vi "test Import Error when No Channels.vi"(8 "error in":errorcluster, 11 "TestCase in":refnum<class "1553 Parameters Import.lvclass">) -> (0 "error out":errorcluster, 3 "TestCase out":refnum<class "1553 Parameters Import.lvclass">)   [LabVIEW 2020, in "1553 Parameters Import.lvclass"]
uses:
  1553 Parameters Import.lvclass
  Shared/BIU Configuration.ctl
  Shared/Address.ctl
  Shared/Major Frame Definition.ctl
  Shared/Minor Frame Definition.ctl
  Shared/Acyclic Frame Definition.ctl
  Shared/Message Definition.ctl
  Shared/Message Type.ctl
  Shared/Terminal Endpoint.ctl
  Shared/Parameter Definition.ctl
  <vilib>/Utility/xml.llb/Write to XML File(string).vi
  <vilib>/addons/_JKI Toolkits/VI Tester/TestCase.llb/TestCase.lvclass
  Import/MIL-STD 1553 Import.lvlib
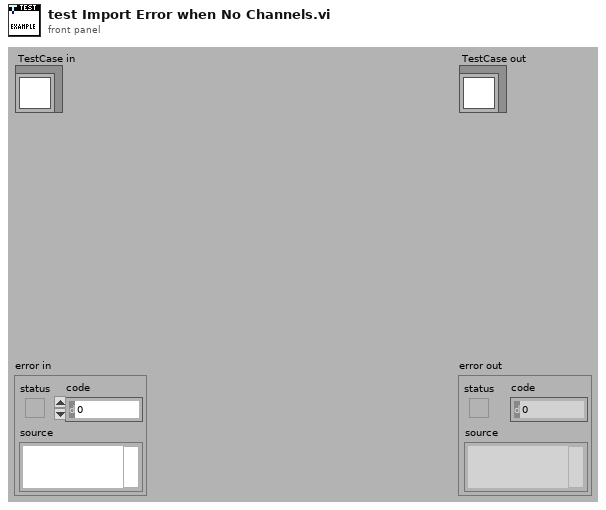
[diagram p1: front panel]
types:
  T1 = typedef "BIU Configuration.ctl" = cluster{"HW channel":u16, "terminal addresses":T2[], "terminal names":string[], "major frames":T3[], "minor frames":T4[], "acyclic frames":T5[], "messages":T6[], "minor frame period (us)":i32}
  T2 = typedef "Address.ctl" = u16
  T3 = typedef "Major Frame Definition.ctl" = cluster{"name":string, "minor frames":string[]}
  T4 = typedef "Minor Frame Definition.ctl" = cluster{"name":string, "messages":string[]}
  T5 = typedef "Acyclic Frame Definition.ctl" = cluster{"name":string, "messages":string[]}
  T6 = typedef "Message Definition.ctl" = cluster{"name":string, "message type":T7, "endpoint Tx":T8, "endpoint Rx":T8, "create timestamp channel":bool, "mode code":u16, "number of words":u16, "parameters":cluster{"name":string, "default value":dbl, "unit":string, "parameter definition":T9}[]}
  T7 = typedef "Message Type.ctl" = string
  T8 = typedef "Terminal Endpoint.ctl" = cluster{"terminal address":T2, "subaddress":T2}
  T9 = typedef "Parameter Definition.ctl" = cluster{"start index":i32, "size (bits)":i32, "encoding":enum16{"BNR", "BCD", "Discrete"}, "signed":bool, "multiplier":dbl, "offset":dbl}
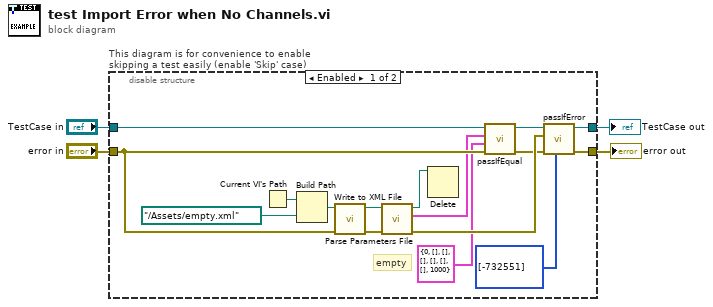
[diagram p0: block diagram]
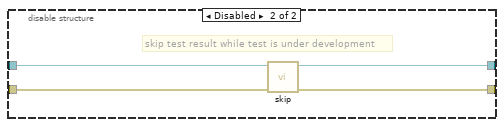
[diagram p2: hidden frame]
diagram:
  n1 = disable-structure "This diagram is for convenience to enable skipping a test easily (enable 'Skip' case)" shown="Enabled" {
    disable-tunnel: "TestCase in" -> [w10 w24]
    disable-tunnel: [w20 w22] -> w1
    disable-tunnel: [w19 w23] -> w3
    disable-tunnel: "error in" -> [w12 w21]
    frame Enabled {
      # "empty"
      n2 = Current VI's Path() -> (path=w8:path)
      n3 = Build Path(base path=w8, name or relative path=path "../Assets/empty.xml") -> (appended path=w18:path)
      n4 = call-poly <vilib>:"Write to XML File.vi"("error in (no error)"=w12, "XML File Path"=w18) -> ("error out"=w16:errorcluster, "XML File Path(duplicate)"=w17:path)  [unwired: 7 in, 1 out]
      n5 = call "Parse Parameters File.vi"("error in"=w16, "path to XML document"=w17) -> ("error out"=w15:errorcluster, "biu configuration"=w6:T1, "path to XML document out"=w9:path)  [unwired: 7 in]
      n6 = Delete(path (use dialog)=w9) -> ()  [unwired: 4 in, 3 out]
      n7 = call-dynamic "passIfEqual.vi"("error in (no error)"=w12, "y"=T1 {"HW channel"=0, "terminal addresses"=[], "terminal names"=[], "major frames"=[], "minor frames"=[], "acyclic frames"=[], "messages"=[], "minor frame period (us)"=1000} ("biu configuration"), "x"=w6, "TestCase in"=w10) -> ("error out"=w13:errorcluster, "TestCase out"=w11:refnum<class "1553 Parameters Import.lvclass">)  [unwired: 6 in]
      n8 = call-dynamic "passIfError.vi"("passing error codes (default = any error code)"=i32[] [-732551], "error in (no error)"=w13, "error"=w15, "TestCase in"=w11) -> ("error out"=w19:errorcluster, "TestCase out"=w20:refnum<class "1553 Parameters Import.lvclass">)  [unwired: 6 in]
    }
    frame Disabled {
      # "skip test result while test is under development"
      n9 = call <vilib>:"skip.vi"("error in (no error)"=w21, "TestCase in"=w24) -> ("error out"=w23:errorcluster, "TestCase out"=w22:refnum<class "1553 Parameters Import.lvclass">)  [unwired: 8 in]
    }
  }
  "error out" <- w3
  "TestCase out" <- w1
